vi "find_midpoint_laser.vi"(3 "Cluster":T1, 4 "reset_tape":bool, 5 "run_time":fxp<+,40,40>) -> (0 "timeOfMidpoint":fxp<+,41,40>, 1 "tape_count":u8, 2 "complete":bool)   [LabVIEW 2018]
uses:
  validated_bool.ctl
  <vilib>/rvi/FXPMathLib/FxpAdd/XNode/nifxpmath_Add.xnode
  <vilib>/rvi/FXPMathLib/FxpMul/XNode/nifxpmath_Multiplier.xnode
  <vilib>/rvi/FXPMathLib/sim/FxpSim.dll
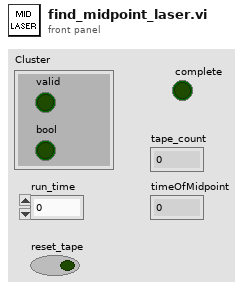
[diagram p1: front panel]
types:
  T1 = typedef "validated_bool.ctl" = cluster{"valid":bool, "bool":bool}
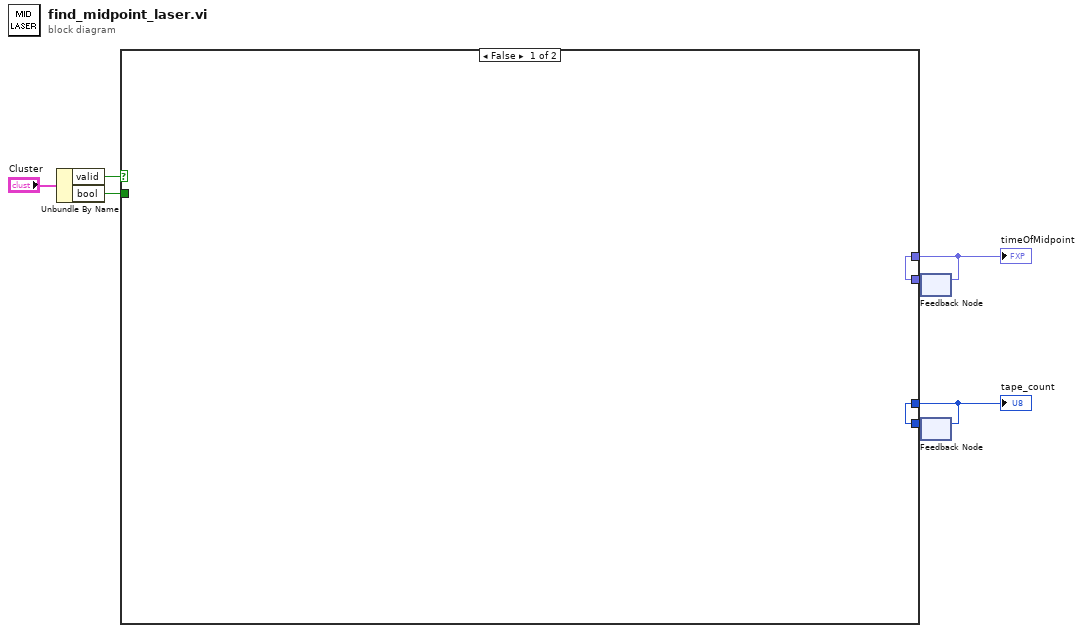
[diagram p0: block diagram]
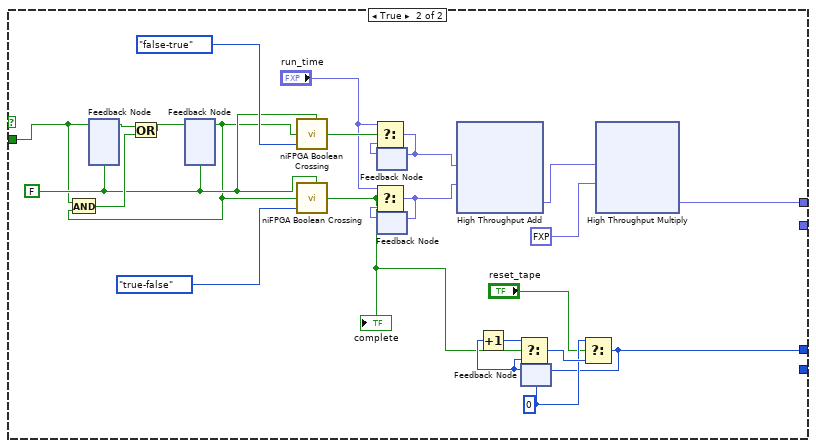
[diagram p2: hidden frame]
diagram:
  n1 = Unbundle By Name("Cluster") -> ("valid"=w7:bool, "bool"=w6:bool)
  n2 = feedback #1() -> (w2:fxp<+,41,40>)  [unwired: 1 in]
  n3 = feedback #2() -> (w1:u8)  [unwired: 1 in]
  n4 = case shown="False" w7 {
    tunnel: w6 -> [_ w18]
    tunnel: [w9 w11] -> w3
    tunnel: [w8 w10] -> w4
    tunnel: w2 -> [w9 _]
    tunnel: w1 -> [w8 _]
    frame False {
    }
    frame True {
      w14 = u8 0
      w30 = FALSE
      n5 = feedback #3(w30) -> (w33:bool)
      n6 = feedback-in #3(w18) -> ()
      n7 = feedback #4(w30) -> (w29:bool)
      n8 = And(x=w18, y=w29) -> (x .and. y?=w32:bool)
      n9 = Or(x=w33, y=w32) -> (x .or. y?=w19:bool)
      n10 = feedback-in #4(w19) -> ()
      n11 = call <vilib>:"niFPGA Boolean Crossing.vi"("input"=w29, "direction"=enum8{"either", "false-true", "true-false"}."false-true", "initialize"=w30) -> ("crossing"=w28:bool)  [unwired: 6 in]
      n12 = call <vilib>:"niFPGA Boolean Crossing.vi"("input"=w29, "direction"=enum8{"either", "false-true", "true-false"}."true-false", "initialize"=w30) -> ("crossing"=w12:bool)  [unwired: 6 in]
      "complete" <- w12
      n13 = feedback #5() -> (w26:fxp<+,40,40>)  [unwired: 1 in]
      n14 = Select(t="run_time", s=w28, f=w26) -> (s? t:f=w23:fxp<+,40,40>)
      n15 = feedback-in #5(w23) -> ()
      n16 = feedback #6() -> (w27:fxp<+,40,40>)  [unwired: 1 in]
      n17 = Select(t="run_time", s=w12, f=w27) -> (s? t:f=w22:fxp<+,40,40>)
      n18 = feedback-in #6(w22) -> ()
      n19 = xnode "High Throughput Add"("x"=w23, "y"=w22) -> ("x+y"=w21:fxp<+,41,41>)
      n20 = feedback #7(w14) -> (w15:u8)
      n21 = Increment(x=w15) -> (x+1=w16:u8)
      n22 = Select(t=w16, s=w12, f=w15) -> (s? t:f=w17:u8)
      n23 = Select(t=w14, s="reset_tape", f=w17) -> (s? t:f=w10:u8)
      n24 = feedback-in #7(w10) -> ()
      n25 = xnode "High Throughput Multiply"("x"=w21, "y"=fxp<+,1,0> 0.5) -> ("x*y"=w11:fxp<+,41,40>)
    }
  }
  "timeOfMidpoint" <- w3
  "tape_count" <- w4
  n26 = feedback-in #1(w3) -> ()
  n27 = feedback-in #2(w4) -> ()
